vi "FrequencyFacade.vi"(0 "Data In":T4, 2 "Display State In":T2, 3 "Container State":T3) -> (6 "Data Out":T4, 7 "Display State Out":T2, 8 "Action":T1)   [LabVIEW 2018, in "Ui.lvlib" / "Frequency.xctl"]
uses:
  Frequency.xctl
  FrequencyData.ctl
  <vilib>/_xctls/Container State.ctl
  FrequencyState.ctl
  <vilib>/_xctls/Action.ctl
  <vilib>/_xctls/XControlSupport.lvlib
panel:
  out "Frequency G":dbl(knob) scale=1.0..100.0
  out "Time":i64
  in  "Frequency":dbl(knob)=1.0 min=1.0 max=100.0 step=1.0 scale=1.0..100.0
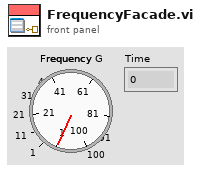
[diagram p1: front panel]
types:
  T1 = typedef "XControlSupport.lvlib/Action.ctl" = cluster{"Data Changed?":bool, "State Changed?":bool, "Action Name":string}
  T2 = typedef "Ui.lvlib/Frequency.xctl/FrequencyState.ctl" = cluster{"Numeric":dbl}
  T3 = typedef "XControlSupport.lvlib/Container State.ctl" = cluster{"Indicator?":bool, "Run Mode?":bool, " Refnum":refnum<vi>}
  T4 = typedef "Ui.lvlib/Frequency.xctl/FrequencyData.ctl" = i64
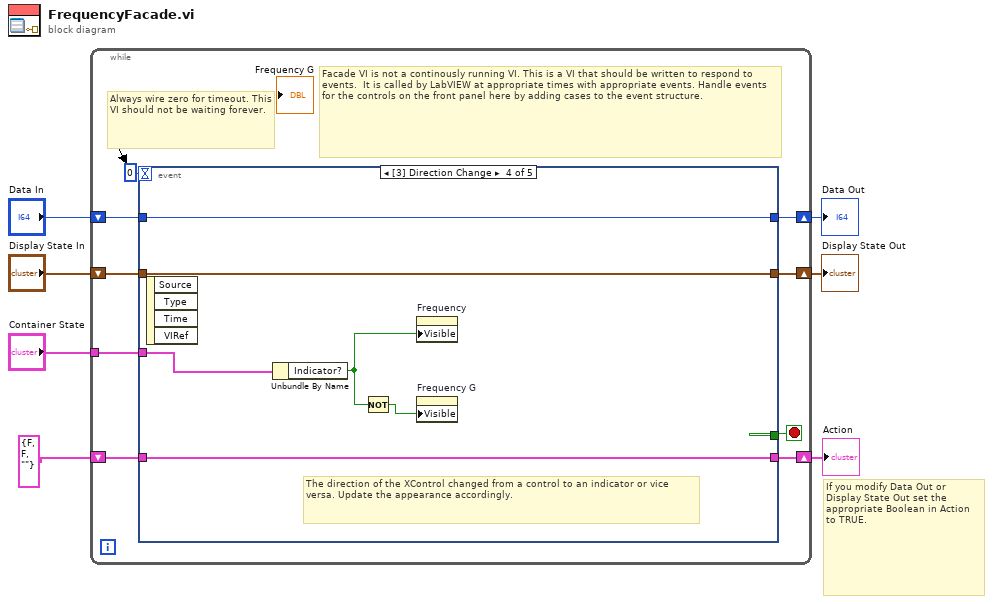
[diagram p0: block diagram]
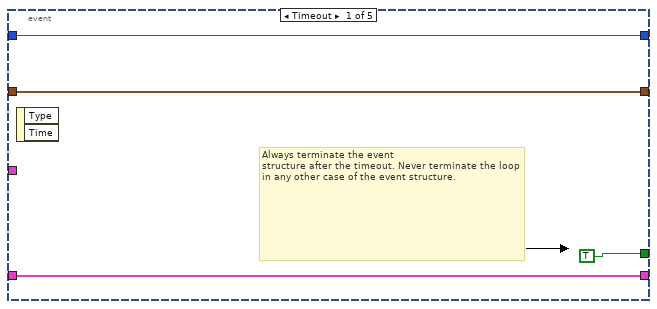
[diagram p2: hidden frame]
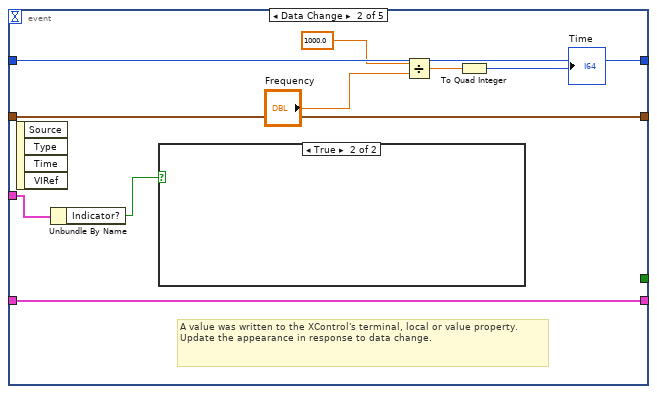
[diagram p3: hidden frame]
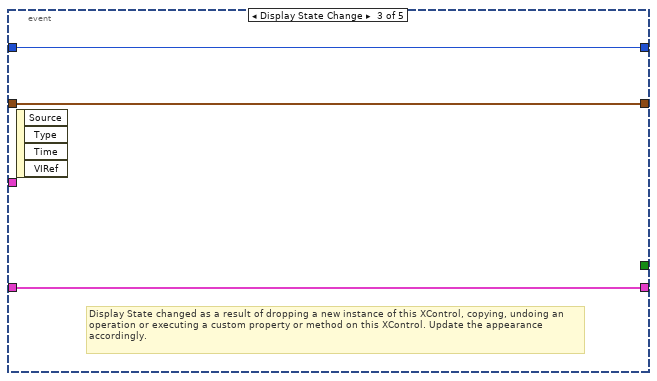
[diagram p5: hidden frame]
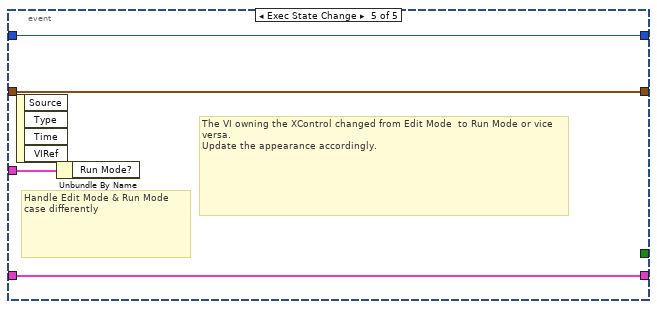
[diagram p6: hidden frame]
diagram:
  # "If you modify Data Out or\nDisplay State Out set the\nappropriate Boolean in Action\nto TRUE."
  n1 = while {
    shift-right: [w15] -> w4
    shift-left: "Display State In" -> [w16]
    tunnel: "Container State" -> [w12]
    shift-right: [w10] -> w7
    shift-left: "Data In" -> [w11]
    shift-right: [w8] -> w2
    shift-left: T1 {"Data Changed?"=FALSE, "State Changed?"=FALSE, "Action Name"=""} ("Action") -> [w9]
    stop <- w14 stop-if-true
    # "Facade VI is not a continously running VI. This is a VI that should be written to respond to events.  It is called by LabVIEW at appropriate times with appropriate events. Handle events for the controls on the front panel here by adding cases to the event structure."
    # "Always wire zero for timeout. This\nVI should not be waiting forever."
    n2 = event shown="[3] Direction Change" {
      selector: _ -> [_ _ _ _ _]
      dyn-events: _ -> [_ _ _ _ _]
      timeout: 0 -> [_ _ _ _ _]
      tunnel: w16 -> [w18 w28 w32 w38 w41]
      tunnel: [w18 w28 w32 w38 w41] -> w15
      tunnel: [TRUE _ _ _ _] -> w14
      tunnel: w12 -> [_ w22 _ w35 w42]
      tunnel: w11 -> [w17 w29 w31 w37 w40]
      tunnel: [w17 w29 w31 w37 w40] -> w10
      tunnel: [w19 w27 w30 w36 w39] -> w8
      tunnel: w9 -> [w19 w27 w30 w36 w39]
      event Timeout {
        # "Always terminate the event\nstructure after the timeout. Never terminate the loop in any other case of the event structure."
        n3 = event-data() -> ()  [unwired: 1 in, 2 out]
      }
      event Data Change {
        # "A value was written to the XControl's terminal, local or value property.\nUpdate the appearance in response to data change."
        n4 = event-data() -> ()  [unwired: 1 in, 4 out]
        n5 = Unbundle By Name(w22) -> ("Indicator?"=w21:bool)
        n6 = case shown="True" w21 {
          frame False {
          }
          frame True {
          }
        }
        n7 = Divide(x=1000.0, y="Frequency") -> (x/y=w23:dbl)
        n8 = To Quad Integer(1:w23) -> (0:→"Time":i64)
      }
      event Display State Change {
        # "Display State changed as a result of dropping a new instance of this XControl, copying, undoing an operation or executing a custom property or method on this XControl. Update the appearance accordingly."
        n9 = event-data() -> ()  [unwired: 1 in, 4 out]
      }
      event Direction Change {
        # "The direction of the XControl changed from a control to an indicator or vice versa. Update the appearance accordingly."
        n10 = event-data() -> ()  [unwired: 1 in, 4 out]
        n11 = Unbundle By Name(w35) -> ("Indicator?"=w33:bool)
        n12 = Not(x=w33) -> (.not. x?=w34:bool)
        n13 = property on="Frequency" class="Knob (strict)"("Visible"=w33) -> ()  [unwired: 2 in, 2 out]
        n14 = property on="Frequency G" class="Knob (strict)"("Visible"=w34) -> ()  [unwired: 2 in, 2 out]
      }
      event Exec State Change {
        # "The VI owning the XControl changed from Edit Mode  to Run Mode or vice versa.\nUpdate the appearance accordingly."
        # "Handle Edit Mode & Run Mode\ncase differently"
        n15 = event-data() -> ()  [unwired: 1 in, 4 out]
        n16 = Unbundle By Name(w42) -> ()  [unwired: 1 out]
      }
    }
  }
  "Display State Out" <- w4
  "Data Out" <- w7
  "Action" <- w2
